vi "SPI Write Byte.vi"() -> ()   [LabVIEW 2020, in "CTI-Scratchpad.lvlib"]
uses:
  CTI-Scratchpad.lvlib
  CTI/SPI Config.ctl
  CTI/SPI Mode.ctl
  CTI/SPI Pins.ctl
  CTI/GPIO Number.ctl
  CTI/Session/Session.lvclass
  CTI/VisaComms/VisaComms.lvclass
  CTI/CTI.lvlib
panel:
  in  "SPI Config":T1={"Mode"=0, "Data Bits"=8, "Pins"={"TX GPIO"=7, "RX GPIO"=4, "SCK GPIO"=6}}
  out "error out":errorcluster
  in  "Baud":u32=500000 format="%.0p"
  in  "Bus":u8
  in  "Port":refnum<visa-resource-name>="COM4"
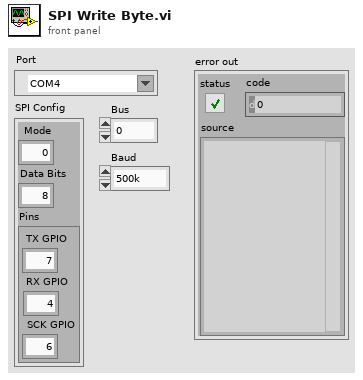
[diagram p1: front panel]
types:
  T1 = typedef "CTI.lvlib/SPI Config.ctl" = cluster{"Mode":T2, "Data Bits":i8, "Pins":T3}
  T2 = typedef "CTI.lvlib/SPI Mode.ctl" = i8
  T3 = typedef "CTI.lvlib/SPI Pins.ctl" = cluster{"TX GPIO":T4, "RX GPIO":T4, "SCK GPIO":T4}
  T4 = typedef "CTI.lvlib/GPIO Number.ctl" = i8
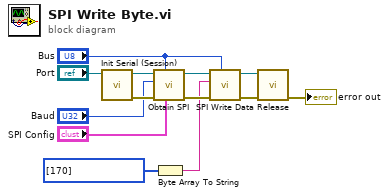
[diagram p0: block diagram]
diagram:
  n1 = call "Init Serial (Session).vi"("VISA resource name in"="Port") -> ("error out"=w12:errorcluster, "Session"=w11:refnum<class "Session.lvclass">)  [unwired: 8 in, 1 out]
  n2 = call "Obtain SPI.vi"("SPI Config"="SPI Config", "SPI #"="Bus", "error in (no error)"=w12, "Baud"="Baud", "Session in"=w11) -> ("error out"=w9:errorcluster, "Session out"=w10:refnum<class "Session.lvclass">)  [unwired: 5 in]
  n3 = Byte Array To String(unsigned byte array=u8[] [170]) -> (string=w3:string)
  n4 = call "SPI Write Data.vi"("SPI #"="Bus", "error in (no error)"=w9, "Data"=w3, "Session in"=w10) -> ("error out"=w7:errorcluster, "Session out"=w6:refnum<class "Session.lvclass">)  [unwired: 6 in]
  n5 = call-dynamic "Release.vi"("error in (no error)"=w7, "Session in"=w6) -> ("error out"=→"error out":errorcluster)  [unwired: 9 in]
